vi "AddChildComponent.vi"(6 "Path":path, 8 "error in (no error)":errorcluster, 9 "Type":string, 10 "ID":string, 11 "head in":refnum<data-value>) -> (0 "error out":errorcluster, 2 "child ref":refnum<data-value>, 3 "head out":refnum<data-value>)   [LabVIEW 2017, in "DirectoryMetadata.lvclass"]
uses:
  DirectoryMetadata.lvclass
  DirectoryMetadata.lvclass/DirectoryMetadata.ctl
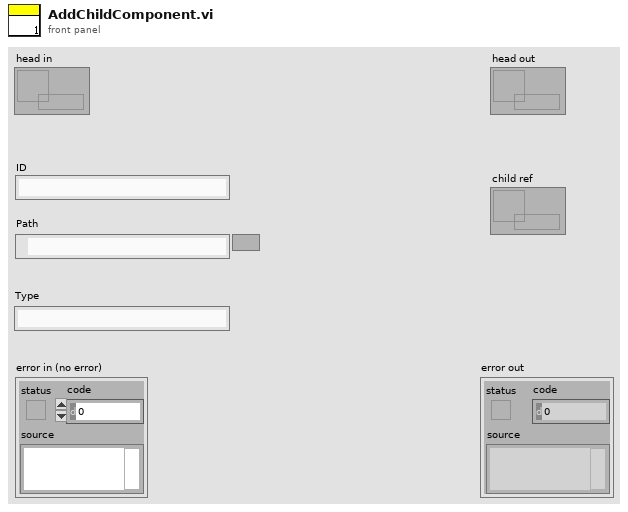
[diagram p1: front panel]
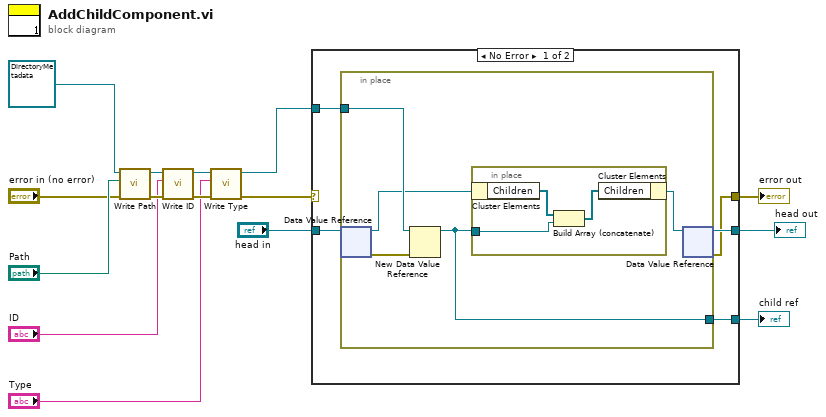
[diagram p0: block diagram]
diagram:
  n1 = call "Write Path.vi"("error in (no error)"="error in (no error)", "Path"="Path", "ClassMetadata in"=refnum<class "DirectoryMetadata.lvclass"> refnum ("Child Ref")) -> ("error out"=w10:errorcluster, "ClassMetadata out"=w13:refnum<class "DirectoryMetadata.lvclass">)  [unwired: 7 in]
  n2 = call "Write ID.vi"("error in (no error)"=w10, "ID"="ID", "ClassMetadata in"=w13) -> ("error out"=w4:errorcluster, "ClassMetadata out"=w7:refnum<class "DirectoryMetadata.lvclass">)  [unwired: 7 in]
  n3 = call "Write Type.vi"("error in (no error)"=w4, "Type"="Type", "ClassMetadata in"=w7) -> ("error out"=w5:errorcluster, "ClassMetadata out"=w6:refnum<class "DirectoryMetadata.lvclass">)  [unwired: 7 in]
  n4 = case shown="No Error" w5 {
    selector: w5 -> [_ w30]
    tunnel: [w16 w30] -> w15
    tunnel: [w17 w29] -> w1
    tunnel: "head in" -> [w18 w29]
    tunnel: w6 -> [w20 _]
    tunnel: [w19 _] -> w9
    frame No Error {
      n5 = in-place {
        in-place-border: w20 -> [w25]
        in-place-border: [w23] -> w19
        n6 = in-place-dvr #1(w18) -> (w24:refnum<class "DirectoryMetadata.lvclass">, w21:errorcluster)
        n7 = New Data Value Reference(data value=w25, error in=w21) -> (data value reference=w23:refnum<data-value>)  [unwired: 1 out]
        n8 = in-place {
          in-place-border: w23 -> [w28]
          n9 = in-place-cluster #2(w24) -> ("Children"=w27:refnum<data-value>[])
          n10 = Build Array (concatenate)(w27, w28) -> (w26:refnum<data-value>[])
          n11 = in-place-cluster #2("Children"=w26) -> (w22:refnum<class "DirectoryMetadata.lvclass">)
        }
        n12 = in-place-dvr #1(w22) -> (w17:refnum<data-value>, w16:errorcluster)
      }
    }
    frame Error {
    }
  }
  "error out" <- w15
  "child ref" <- w9
  "head out" <- w1
